vi "Build greater unit test strings.vi"(11 "all rows":string[](array[string])) -> (1 "Chaîne 4":string, 2 "Chaîne":string, 3 "Chaîne 2":string, 4 "Chaîne 3":string, 5 "Numérique":i32, 6 "offset past number":i32)   [LabVIEW 2021]
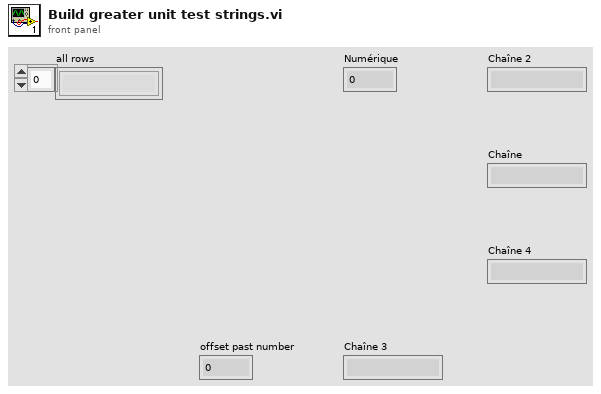
[diagram p1: front panel]
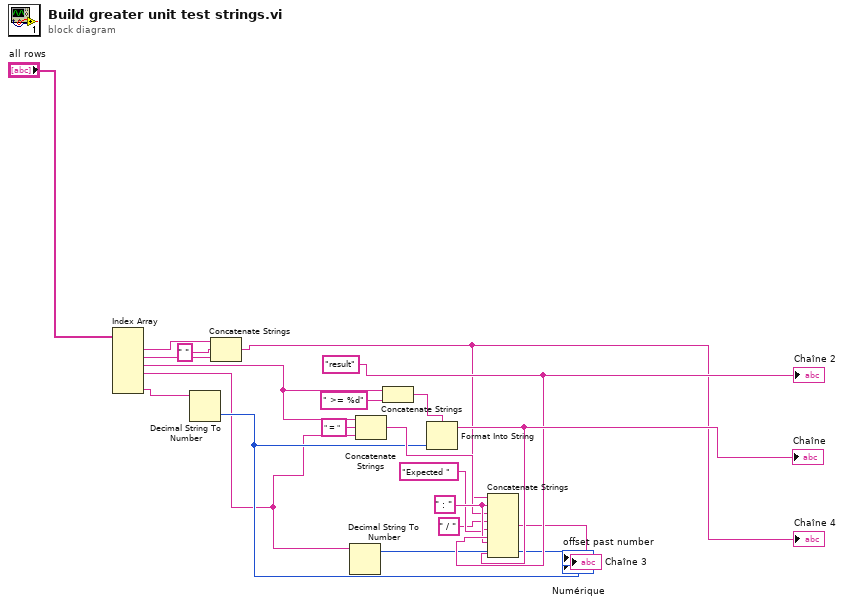
[diagram p0: block diagram]
diagram:
  w16 = " : " ("chaîne")
  w17 = "result"
  n1 = Index Array ("Indexer un tableau")(array="all rows") -> (element #1=w2:string, element #2=w4:string, element #3=w6:string, element #4=w7:string, element #6=w8:string)  [unwired: 6 in, 1 out]
  n2 = Decimal String To Number ("Chaîne décimale en nombre")(string=w8) -> (number=w9:i32)  [unwired: 2 in, 1 out]
  "Numérique" <- w9
  n3 = Concatenate Strings ("Concaténer des chaînes")(w2, " " ("chaîne"), w4) -> (w5:string)
  "Chaîne 4" <- w5
  n4 = Decimal String To Number(string=w7) -> (offset past number=→"offset past number":i32)  [unwired: 2 in, 1 out]
  n5 = Concatenate Strings(w6, " = " ("chaîne"), w7) -> (w14:string)
  n6 = Concatenate Strings(w6, " >= %d" ("chaîne")) -> (w19:string)
  n7 = Format Into String(format string=w19, w9) -> (resulting string=w20:string)  [unwired: 2 in, 1 out]
  "Chaîne" <- w20
  n8 = Concatenate Strings(w5, w16, w14, " / " ("chaîne"), "Expected " ("chaîne"), w17, w16, w20) -> (→"Chaîne 3":string)
  "Chaîne 2" <- w17
